vi "GUI DC meter setup.vi"(11 "DC meter":T2={"DC meter type"=enum."H/A/K 3458", "DC meter VISA"="", "NPLC"=10.0, "No of readings"=3.0}) -> (3 "DC meter out":T2={"DC meter type"=enum."H/A/K 3458", "DC meter VISA"="", "NPLC"=10.0, "No of readings"=3.0})   [LabVIEW 2020]
doc: "Use this template to build a producer/consumer design pattern with events to produce queue items. Use this design pattern instead of the User Interface Event Handler pattern for user interfaces when you want to execute code asynchronously in response to an event without slowing the user interface responsiveness."
uses:
  General DC meter/Type definitions/DC meter.ctl
  General DC meter/Type definitions/DC meter type.ctl
  <vilib>/Utility/error.llb/DialogType.ctl
  <vilib>/Utility/error.llb/Error Cluster From Error Code.vi
  <vilib>/ErrorRing/Error Ring.xnode
  external libraries/varilib/varilib.lvlib
panel:
  in  "NPLC":dbl=10.0
  in  "Number of readings":dbl=3.0
  in  "DC meter type":T1
  in  "NI DAQ help":string="NI DAQ will be set to generate 2 signals:\n\n- 5 MHz signal at output /ctr_1. Signal is used to synchronize generator and digitizer PXI 5922 using input CLK_IN.\n\n- Trigger signal at output /ctr_0."
  in  "VISA":refnum<visa-resource-name>
  out "gui_elements":refnum<vi>[](array[refnum])
  out "Status":string
  in  "save_and_quit":bool
  in  "test":bool
  in  "cancel":bool
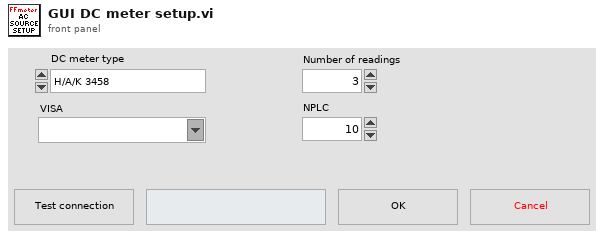
[diagram p1: front panel]
types:
  T1 = typedef "DC meter type.ctl" = enum16{"H/A/K 3458", "FLuke 8508A", "dummy"}
  T2 = typedef "DC meter.ctl" = cluster{"DC meter type":T1, "DC meter VISA":refnum<visa-resource-name>, "NPLC":dbl, "No of readings":dbl}
  T3 = typedef "DialogType.ctl" = u16
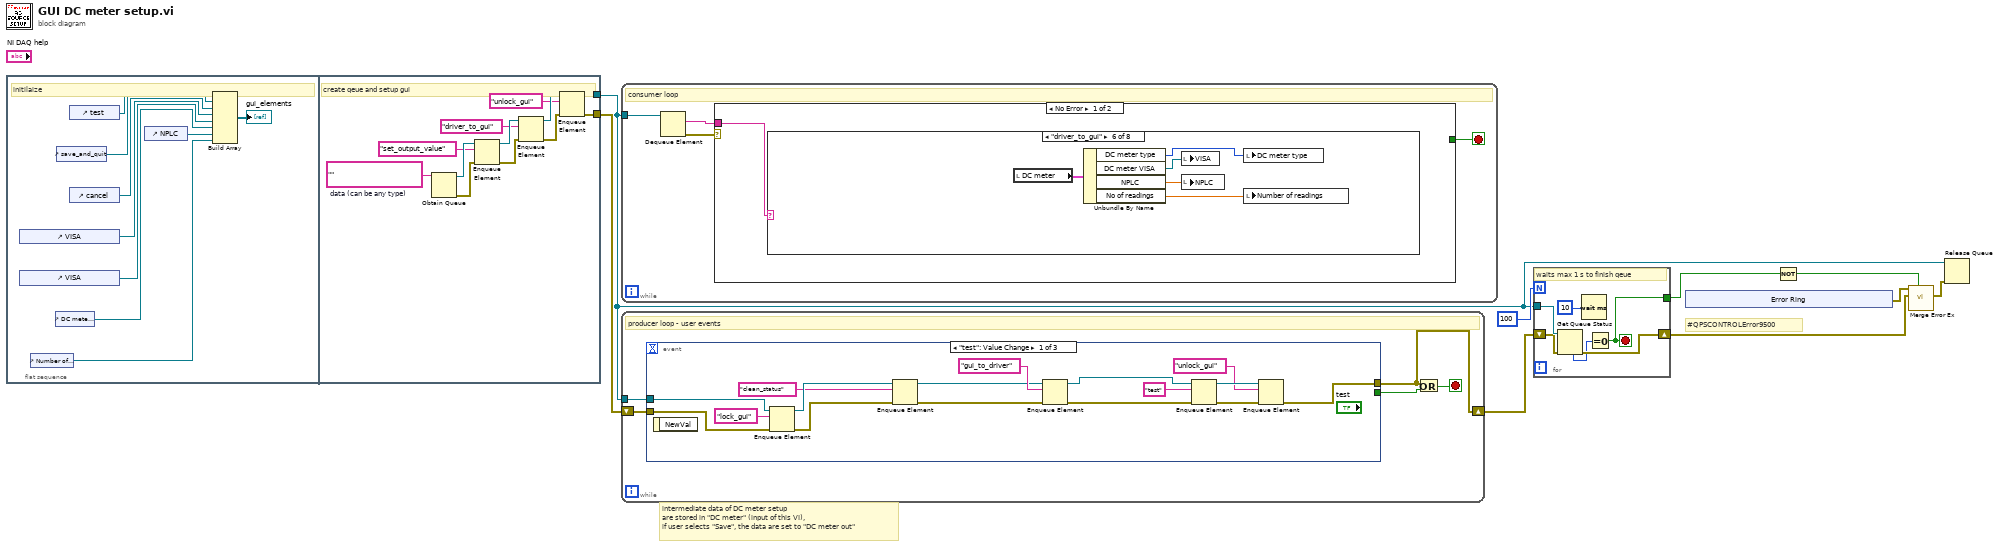
[diagram p0: block diagram]
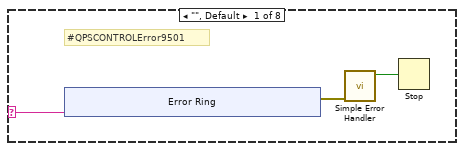
[diagram p2: hidden frame]
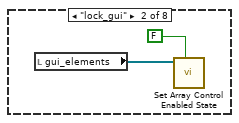
[diagram p3: hidden frame]
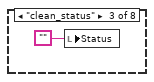
[diagram p4: hidden frame]
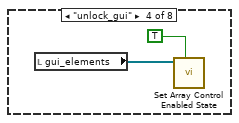
[diagram p5: hidden frame]
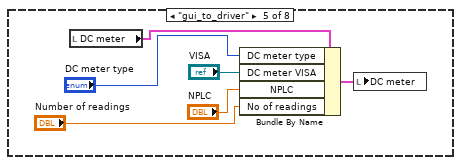
[diagram p6: hidden frame]
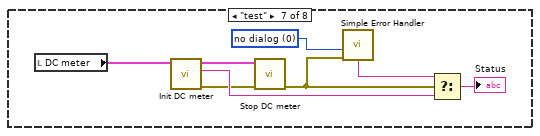
[diagram p7: hidden frame]
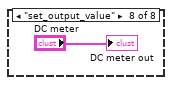
[diagram p8: hidden frame]
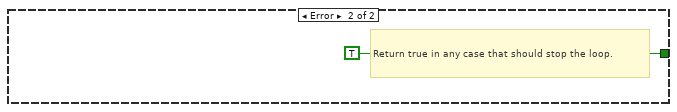
[diagram p9: hidden frame]
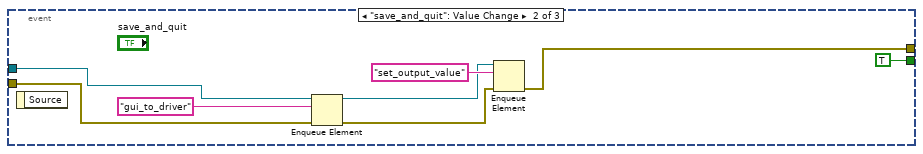
[diagram p10: hidden frame]
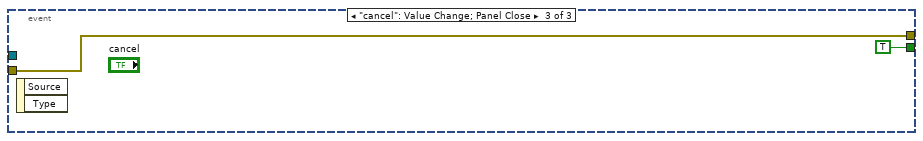
[diagram p11: hidden frame]
diagram:
  # "#QPSCONTROLError9500"
  # "intermediate data of DC meter setup\nare stored in \"DC meter\" (input of this VI),\nif user selects \"Save\", the data are set to \"DC meter out\""
  n1 = flat-sequence {
    tunnel: [w21] -> w2
    tunnel: [w19] -> w1
    frame #0 {
      # "initilaize"
      n2 = control-ref of="VISA"() -> (w12:refnum<vi>)
      n3 = control-ref of="VISA"() -> (w14:refnum<vi>)
      n4 = control-ref of="Number of readings"() -> (w10:refnum<vi>)
      n5 = control-ref of="DC meter type"() -> (w13:refnum<vi>)
      n6 = control-ref of="save_and_quit"() -> (w17:refnum<vi>)
      n7 = control-ref of="test"() -> (w18:refnum<vi>)
      n8 = control-ref of="cancel"() -> (w16:refnum<vi>)
      n9 = control-ref of="NPLC"() -> (w11:refnum<vi>)
      n10 = Build Array(w18, w17, w16, w12, w14, w13, w11, w10) -> (→"gui_elements":refnum<vi>[])
    }
    frame #1 {
      w20 = ""  # data (can be any type)
      # "create qeue and setup gui"
      n11 = Obtain Queue(element data type=w20) -> (queue out=w25:refnum<queue>, error out=w27:errorcluster)  [unwired: 4 in, 1 out]
      n12 = Enqueue Element(queue=w25, element="set_output_value", error in (no error)=w27) -> (queue out=w26:refnum<queue>, error out=w28:errorcluster)  [unwired: 1 in, 1 out]
      n13 = Enqueue Element(queue=w26, element="driver_to_gui", error in (no error)=w28) -> (queue out=w30:refnum<queue>, error out=w29:errorcluster)  [unwired: 1 in, 1 out]
      n14 = Enqueue Element(queue=w30, element="unlock_gui", error in (no error)=w29) -> (queue out=w21:refnum<queue>, error out=w19:errorcluster)  [unwired: 1 in, 1 out]
    }
  }
  n15 = while {
    tunnel: w2 -> [w34]
    stop <- w31 stop-if-true
    # "consumer loop"
    n16 = Dequeue Element(queue=w34) -> (element=w32:string, error out=w33:errorcluster)  [unwired: 2 in, 2 out]
    n17 = case shown="No Error" w33 {
      tunnel: w32 -> [w35 _]
      tunnel: [_ TRUE] -> w31
      frame No Error {
        n18 = case shown="\"driver_to_gui\"" w35 {
          selector: w35 -> [w36 _ _ _ _ _ _ _]
          frame "", Default {
            # "#QPSCONTROLError9501"
            n19 = xnode "Error Ring"("parameter 0"=w36) -> ("error out"=w38:errorcluster)
            n20 = call <vilib>:"Simple Error Handler.vi"("error in (no error)"=w38) -> ("error?"=w37:bool)  [unwired: 4 in, 4 out]
            n21 = Stop(stop? (T)=w37) -> ()
          }
          frame "lock_gui" {
            n22 = local read "gui_elements"() -> (w47:refnum<vi>[])
            n23 = call "Set Array Control Enabled State.vi"("enabled (T)"=FALSE, "reference array in"=w47) -> ()  [unwired: 8 in, 2 out]
          }
          frame "clean_status" {
            n24 = local write "Status"("") -> ()
          }
          frame "unlock_gui" {
            n25 = local read "gui_elements"() -> (w50:refnum<vi>[])
            n26 = call "Set Array Control Enabled State.vi"("enabled (T)"=TRUE, "reference array in"=w50) -> ()  [unwired: 8 in, 2 out]
          }
          frame "gui_to_driver" {
            n27 = local read "DC meter"() -> (w55:T2)
            n28 = Bundle By Name(cluster=w55, "DC meter type"="DC meter type", "DC meter VISA"="VISA", "NPLC"="NPLC", "No of readings"="Number of readings") -> (w56:T2)
            n29 = local write "DC meter"(w56) -> ()
          }
          frame "driver_to_gui" {
            n30 = local read "DC meter"() -> (w61:T2)
            n31 = Unbundle By Name(w61) -> ("DC meter type"=w60:T1, "DC meter VISA"=w59:refnum<visa-resource-name>, "NPLC"=w58:dbl, "No of readings"=w57:dbl)
            n32 = local write "VISA"(w59) -> ()
            n33 = local write "NPLC"(w58) -> ()
            n34 = local write "DC meter type"(w60) -> ()
            n35 = local write "Number of readings"(w57) -> ()
          }
          frame "test" {
            w69 = T3 0 items=["no dialog", "OK message", "continue or stop message", "OK message + warnings", "continue/stop + warnings"] ("type of dialog (OK msg:1)")
            n36 = local read "DC meter"() -> (w66:T2)
            n37 = call "Init DC meter.vi"("DC meter"=w66) -> ("error out"=w63:errorcluster, "Init status"=w65:string, "DC meter out"=w62:T2)  [unwired: 8 in]
            n38 = call "Stop DC meter.vi"("error in (no error)"=w63, "DC meter"=w62) -> ("error out"=w64:errorcluster)  [unwired: 8 in, 1 out]
            n39 = call <vilib>:"Simple Error Handler.vi"("type of dialog (OK msg:1)"=w69, "error in (no error)"=w64) -> ("message"=w68:string)  [unwired: 3 in, 4 out]
            n40 = Select(t=w68, s=w64, f=w65) -> (s? t:f=→"Status":string)
          }
          frame "set_output_value" {
            "DC meter out" <- "DC meter"
          }
        }
      }
      frame Error {
        # "Return true in any case that should stop the loop."
      }
    }
  }
  n41 = while {
    shift-right: [w72] -> w5
    shift-left: w1 -> [w75]
    tunnel: w2 -> [w76]
    stop <- w73 stop-if-true
    # "producer loop - user events"
    n42 = event shown="[0] \"test\": Value Change" {
      selector: _ -> [_ _ _]
      dyn-events: _ -> [_ _ _]
      timeout: _ -> [_ _ _]
      tunnel: w76 -> [w83 w97 _]
      tunnel: w75 -> [w84 w94 w102]
      tunnel: [w87 w93 w102] -> w72
      tunnel: [_ TRUE ("cancel") TRUE ("cancel")] -> w74
      event "test": Value Change {
        n43 = event-data() -> ()  [unwired: 1 in, 1 out]
        n44 = Enqueue Element(queue=w83, element="lock_gui", error in (no error)=w84) -> (queue out=w80:refnum<queue>, error out=w81:errorcluster)  [unwired: 1 in, 1 out]
        n45 = Enqueue Element(queue=w80, element="clean_status", error in (no error)=w81) -> (queue out=w78:refnum<queue>, error out=w79:errorcluster)  [unwired: 1 in, 1 out]
        n46 = Enqueue Element(queue=w78, element="gui_to_driver", error in (no error)=w79) -> (queue out=w90:refnum<queue>, error out=w91:errorcluster)  [unwired: 1 in, 1 out]
        n47 = Enqueue Element(queue=w90, element="test", error in (no error)=w91) -> (queue out=w86:refnum<queue>, error out=w88:errorcluster)  [unwired: 1 in, 1 out]
        n48 = Enqueue Element(queue=w86, element="unlock_gui", error in (no error)=w88) -> (error out=w87:errorcluster)  [unwired: 1 in, 2 out]
      }
      event "save_and_quit": Value Change {
        n49 = event-data() -> ()  [unwired: 1 in, 1 out]
        n50 = Enqueue Element(queue=w97, element="gui_to_driver", error in (no error)=w94) -> (queue out=w96:refnum<queue>, error out=w95:errorcluster)  [unwired: 1 in, 1 out]
        n51 = Enqueue Element(queue=w96, element="set_output_value", error in (no error)=w95) -> (error out=w93:errorcluster)  [unwired: 1 in, 2 out]
      }
      event "cancel": Value Change; Panel Close {
        n52 = event-data() -> ()  [unwired: 1 in, 2 out]
      }
    }
    n53 = Or(x=w72, y=w74) -> (x .or. y?=w73:bool)
  }
  n54 = for {
    N: 100 -> [_]
    tunnel: w2 -> [w108]
    shift-right: [w106] -> w6
    shift-left: w5 -> [w107]
    tunnel: [w103] -> w3
    stop <- w103 stop-if-true
    # "waits max 1 s to finish qeue"
    n55 = Get Queue Status(queue=w108, error in (no error)=w107) -> (error out=w106:errorcluster, # elements in queue=w104:i32)  [unwired: 1 in, 6 out]
    n56 = Wait (ms)(milliseconds to wait=u32 10) -> ()  [unwired: 1 out]
    n57 = Equal To 0?(x=w104) -> (x = 0?=w103:bool)
  }
  n58 = xnode "Error Ring"() -> ("error out"=w7:errorcluster)
  n59 = Not(x=w3) -> (.not. x?=w8:bool)
  n60 = call "Merge Error Ex.vi"("Is error? (False)"=w8, "main error in (no error)"=w6, "second error in"=w7) -> ("error out"=w4:errorcluster)  [unwired: 8 in]
  n61 = Release Queue(queue=w2, error in (no error)=w4) -> ()  [unwired: 1 in, 3 out]
